vi "adc_basic_fetch_data.vi"(2 "CCS Base Folder 2":path=path "C:/ti/ccs930/ccs/ccs_base", 3 "CCXML File (target configuration)":path=path "D:/Projects/C2000/Grande/c2000_topogrande_avv/bitfield-submodule/common/targetConfigs/TMS320F280039C.ccxml", 4 "program file":path=path "D:/Projects/C2000/Grande/c2000_topogrande_avv/testcases_non_avv/ADC/adc_off-gain/Debug/topog_adc_off-gain.out", 5 "error in (no error)":errorcluster) -> (16 "AvgCode":dbl, 19 "error out":errorcluster)   [LabVIEW 2019]
uses:
  <userlib>/_TI-LA/Reusable/CCS/APIs/Data/Polymorphics/Write Data To Symbol - U16.vi
  <userlib>/_TI-LA/Reusable/CCS/APIs/CCS.lvlib
  <vilib>/Analysis/NI_AALBase.lvlib
panel:
  out "Programed":bool
  out "standard deviation":dbl format="%0.2f"
  out "mean":dbl format="%0.2f"
  in  "Repeat":bool
  in  "stop":bool
  in  "Data_File":path=path "D:/Projects/C2000/Grande/Data/ADC/Offset_Gain/New Text Document.txt"
  out "Waveform Graph":u16[](graph)
  out "Read Data[]":u16[](array[numeric]) format="%#.0f"
  # "C:\\ti\\ccsv6\\ccs_base"
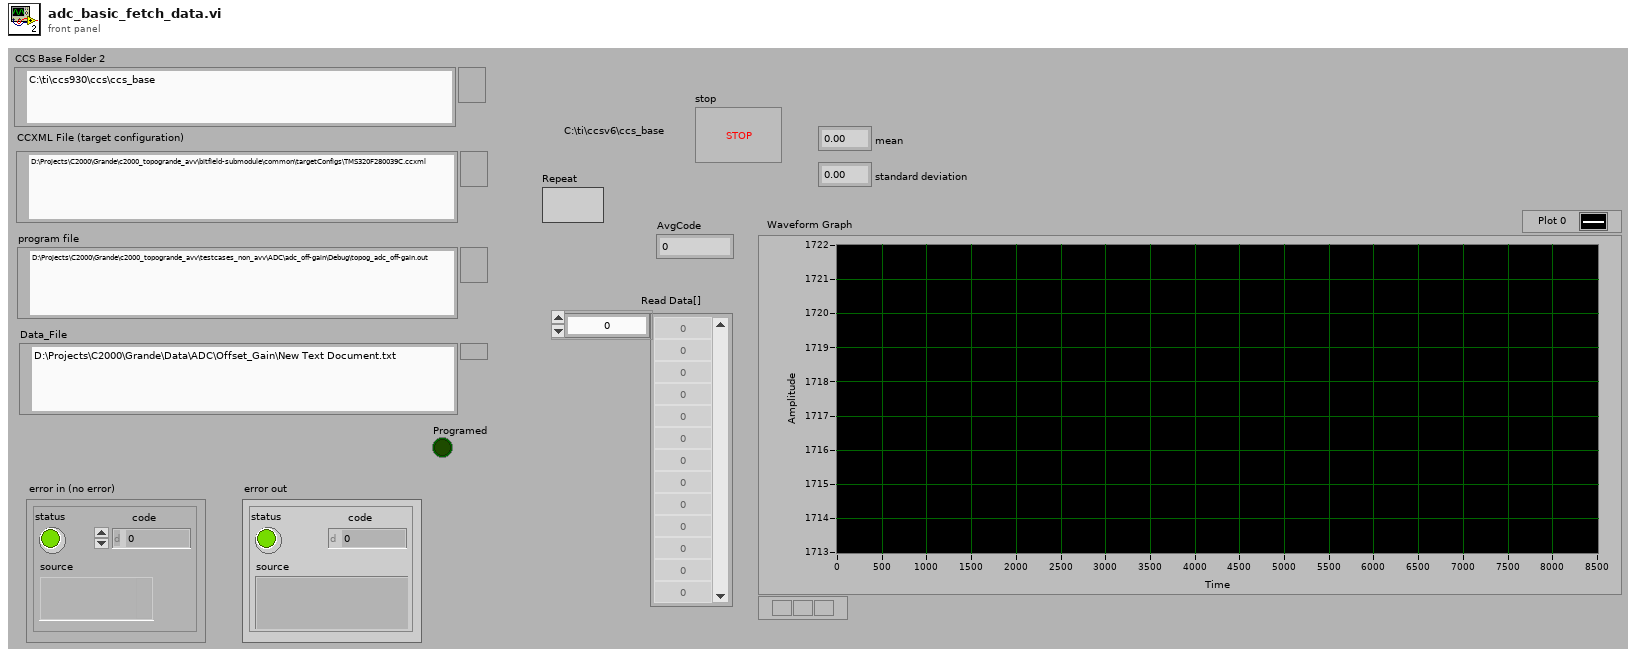
[diagram p1: front panel]
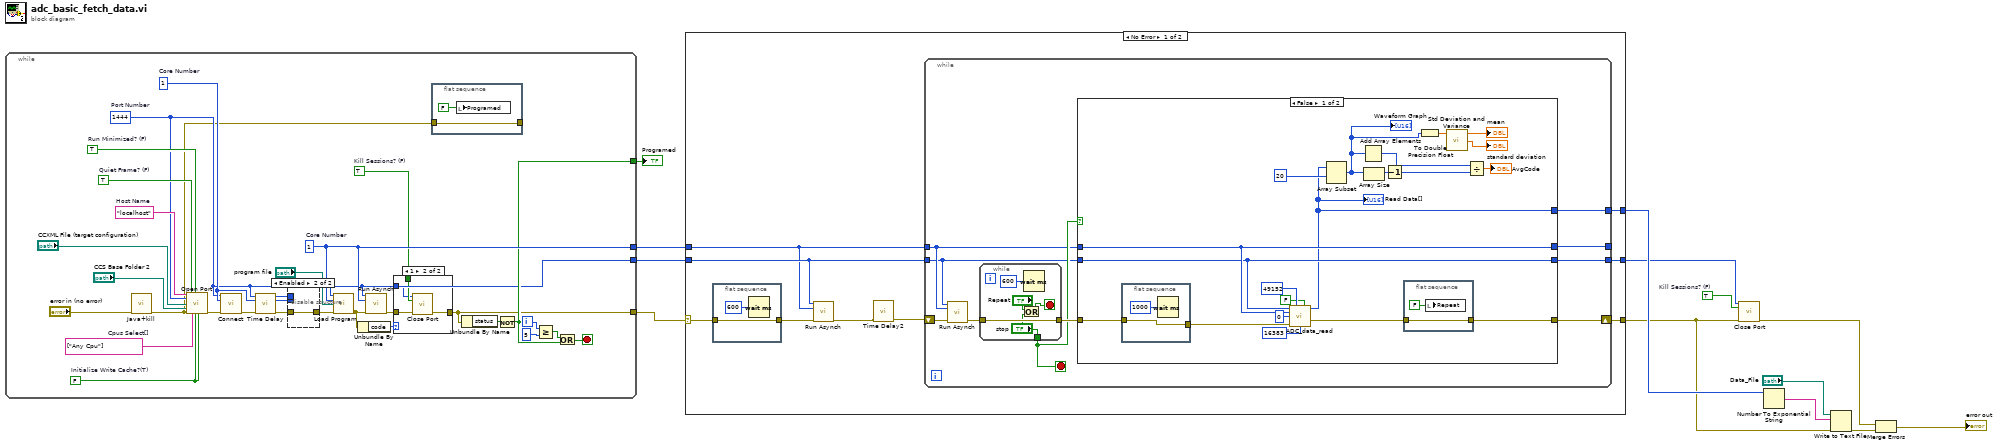
[diagram p0: block diagram]
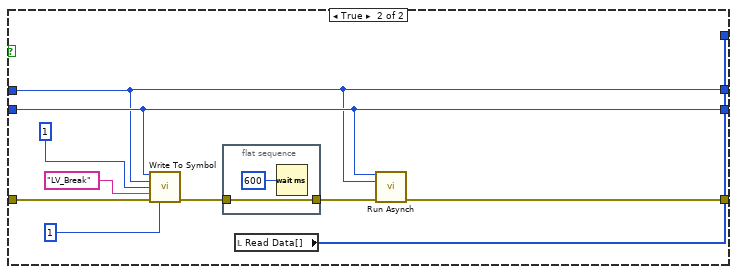
[diagram p2: hidden frame]
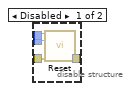
[diagram p5: hidden frame]
diagram:
  w13 = TRUE  # Kill Sessions? (F)
  n1 = while {
    tunnel: [w16] -> w2
    tunnel: [w15] -> w6
    tunnel: [w25] -> w5
    tunnel: [w21] -> w1
    i -> [w27]
    stop <- w28 stop-if-true
    w18 = TRUE  # Kill Sessions? (F)
    w25 = u16 1  # Core Number
    w26 = u16 1  # Core Number
    w34 = FALSE  # Initialize Write Cache?(T)
    w35 = string[] ["Any Cpu"]  # Cpus Select[]
    w36 = TRUE  # Run Minimized? (F)
    w37 = TRUE  # Quiet Frame? (F)
    w15 = u16 1444  # Port Number
    w40 = "localhost"  # Host Name
    n2 = call "Java+kill.vi"("error in (no error)"="error in (no error)") -> ("error out"=w14:errorcluster)  [unwired: 10 in]
    n3 = call <userlib>:"Open Port.vi"("Host Name"=w40, "Port Number"=w15, "CCXML File"="CCXML File (target configuration)", "CCS Base Folder"="CCS Base Folder 2", "error in"=w14, "Quiet Frame? (F)"=w37, "Cpus Select[]"=w35, "Run Minimized? (F)"=w36, "Initialize Write Cache?(T)"=w34, "Initialize Symbol Cache?(T)"=w34) -> ("error out"=w41:errorcluster)  [unwired: 7 in, 2 out]
    n4 = call <userlib>:"Connect.vi"("Port Number"=w15, "Core Number"=w26, "error in"=w41) -> ("error out"=w23:errorcluster)  [unwired: 10 in, 2 out]
    n5 = call "Time Delay"("error in (no error)"=w23) -> ("error out"=w22:errorcluster)  [unwired: 10 in]
    n6 = disable-structure shown="Enabled" {
      disable-tunnel: w22 -> [w52 w53]
      disable-tunnel: [w51 w53] -> w33
      disable-tunnel: w26 -> [w50 _]
      disable-tunnel: w15 -> [w49 _]
      frame Disabled {
        n7 = call <userlib>:"Reset.vi"("Port Number"=w49, "Core Number"=w50, "error in"=w52) -> ("error out"=w51:errorcluster)  [unwired: 10 in, 2 out]
      }
      frame Enabled {
      }
    }
    n8 = call <userlib>:"Load Program.vi"("Port Number"=w15, "Core Number"=w25, "Program File Path"="program file", "error in"=w33) -> ("error out"=w20:errorcluster)  [unwired: 7 in, 4 out]
    n9 = Unbundle By Name(w20) -> ("code"=w19:i32)
    n10 = call <userlib>:"Run Asynch.vi"("Port Number"=w15, "Core Number"=w25, "error in"=w20) -> ("error out"=w17:errorcluster)  [unwired: 10 in, 2 out]
    n11 = case shown="1" w19 {
      tunnel: w18 -> [_ w48]
      tunnel: w17 -> [w44 w47]
      tunnel: [w44 w46] -> w16
      tunnel: w15 -> [_ w45]
      frame Default {
      }
      frame 1 {
        n12 = call <userlib>:"Close Port.vi"("Port Number"=w45, "Kill Sessions? (F)"=w48, "error in"=w47) -> ("error out"=w46:errorcluster)  [unwired: 10 in, 2 out]
      }
    }
    n13 = flat-sequence {
      tunnel: w14 -> [w42]
      tunnel: [w42] -> _
      frame #0 {
        n14 = local write "Programed"(FALSE ("Repeat")) -> ()
      }
    }
    n15 = Unbundle By Name(w16) -> ("status"=w29:bool)
    n16 = Not(x=w29) -> (.not. x?=w21:bool)
    n17 = Greater Or Equal?(x=w27, y=5) -> (x >= y?=w31:bool)
    n18 = Or(x=w31, y=w21) -> (x .or. y?=w28:bool)
  }
  "Programed" <- w1
  n19 = case shown="No Error" w2 {
    selector: w2 -> [w56 w116]
    tunnel: [w62 _] -> w12
    tunnel: w6 -> [w60 _]
    tunnel: w5 -> [w59 _]
    tunnel: [w58 _] -> w4
    tunnel: [w57 w116] -> w3
    frame No Error {
      n20 = flat-sequence {
        tunnel: [w114] -> w61
        tunnel: w56 -> [w114]
        frame #0 {
          n21 = Wait (ms)(milliseconds to wait=u32 600) -> ()  [unwired: 1 out]
        }
      }
      n22 = call <userlib>:"Run Asynch.vi"("Port Number"=w60, "Core Number"=w59, "error in"=w61) -> ("error out"=w55:errorcluster)  [unwired: 10 in, 2 out]
      n23 = call "Time Delay2"("error in (no error)"=w55) -> ("error out"=w54:errorcluster)  [unwired: 10 in]
      n24 = while {
        tunnel: w59 -> [w65]
        tunnel: w60 -> [w64]
        tunnel: [w72] -> w62
        shift-right: [w71] -> w57
        shift-left: w54 -> [w66]
        tunnel: [w67] -> w58
        tunnel: [w68] -> _
        stop <- w69 stop-if-true
        n25 = call <userlib>:"Run Asynch.vi"("Port Number"=w64, "Core Number"=w65, "error in"=w66) -> ("error out"=w63:errorcluster)  [unwired: 10 in, 2 out]
        n26 = while {
          tunnel: [w112] -> w70
          tunnel: w63 -> [w112]
          tunnel: ["stop"] -> w69
          stop <- w111 stop-if-true
          n27 = Or(x="Repeat", y="stop") -> (x .or. y?=w111:bool)
          n28 = Wait (ms)(milliseconds to wait=u32 600) -> ()  [unwired: 1 out]
        }
        n29 = case shown="False" w69 {
          tunnel: w65 -> [w88 w102]
          tunnel: [w78 w106] -> w72
          tunnel: [w79 w105] -> w71
          tunnel: w64 -> [w87 w103]
          tunnel: w70 -> [w80 w104]
          tunnel: [w88 w102] -> w68
          tunnel: [w87 w103] -> w67
          frame False {
            n30 = flat-sequence {
              tunnel: w80 -> [w95]
              tunnel: [w95] -> w89
              frame #0 {
                n31 = Wait (ms)(milliseconds to wait=u32 1000) -> ()  [unwired: 1 out]
              }
            }
            n32 = call "ADC_data_read.vi"("Port Number"=w87, "Address"=u32 49152, "Read_AVG ?"=FALSE, "Core Number"=w88, "Page"=0, "error in (no error)"=w89, "Lv_Samples"=u32 16383) -> ("Read Data[]"=w78:u16[], "error out"=w77:errorcluster)  [unwired: 6 in, 1 out]
            "Read Data[]" <- w78
            n33 = Array Subset(array=w78, index=20) -> (w85:u16[])  [unwired: 1 in]
            "Waveform Graph" <- w85
            n34 = Add Array Elements(numeric array=w85) -> (sum=w92:u16)
            n35 = Array Size(array=w85) -> (size(s)=w82:i32)
            n36 = Decrement(x=w82) -> (x-1=w81:i32)
            n37 = flat-sequence {
              tunnel: w77 -> [w93]
              tunnel: [w93] -> w79
              frame #0 {
                n38 = local write "Repeat"(FALSE ("Repeat")) -> ()
              }
            }
            n39 = To Double Precision Float(number=w85) -> (double precision float=w86:dbl[])
            n40 = call <vilib>:"Std Deviation and Variance.vi"("X"=w86) -> ("mean"=→"mean":dbl, "standard deviation"=→"standard deviation":dbl)  [unwired: 1 in, 1 out]
            n41 = Divide(x=w92, y=w81) -> (x/y=→"AvgCode":dbl)
          }
          frame True {
            n42 = call-poly <userlib>:"Write To Symbol.vi"("Port Number"=w103, "Core Number"=w102, "Page"=1, "Symbol Name"="LV_Break", "error in"=w104, "Write Data"=u16 1) -> ("error out"=w98:errorcluster)  [unwired: 7 in, 2 out]
            n43 = flat-sequence {
              tunnel: [w107] -> w97
              tunnel: w98 -> [w107]
              frame #0 {
                n44 = Wait (ms)(milliseconds to wait=u32 600) -> ()  [unwired: 1 out]
              }
            }
            n45 = local read "Read Data[]"() -> (w106:u16[])
            n46 = call <userlib>:"Run Asynch.vi"("Port Number"=w103, "Core Number"=w102, "error in"=w97) -> ("error out"=w105:errorcluster)  [unwired: 10 in, 2 out]
          }
        }
      }
    }
    frame Error {
    }
  }
  n47 = call <userlib>:"Close Port.vi"("Port Number"=w4, "Kill Sessions? (F)"=w13, "error in"=w3) -> ("error out"=w8:errorcluster)  [unwired: 10 in, 2 out]
  n48 = Number To Exponential String(number=w12) -> (E-format string=w11:string[])  [unwired: 3 in]
  n49 = Write to Text File(file (use dialog)="Data_File", text=w11, error in=w3) -> (error out=w9:errorcluster)  [unwired: 1 in, 2 out]
  n50 = Merge Errors(w8, w9) -> (→"error out":errorcluster)
